vi "JSON Error to Error Cluster.vi"(8 "error in (no error)":errorcluster, 10 "headers":string, 11 "JSON string":string) -> (0 "error out":errorcluster)   [LabVIEW 2013, in "Particle API.lvlib"]
uses:
  Particle API.lvlib
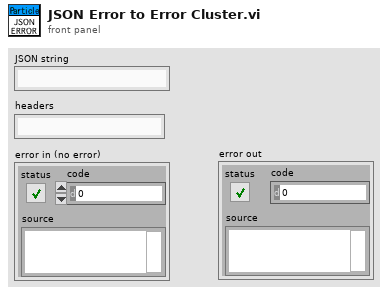
[diagram p1: front panel]
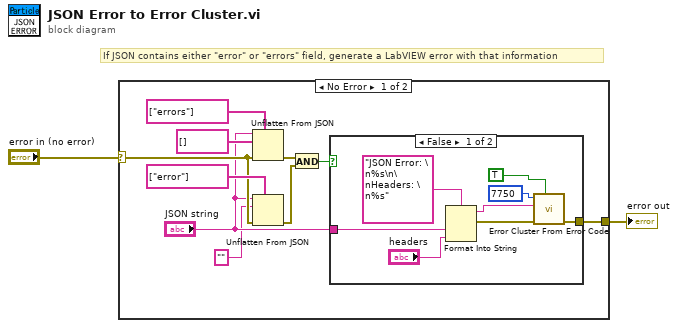
[diagram p0: block diagram]
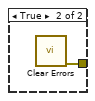
[diagram p2: hidden frame]
diagram:
  # "If JSON contains either \"error\" or \"errors\" field, generate a LabVIEW error with that information"
  n1 = case shown="No Error" "error in (no error)" {
    selector: "error in (no error)" -> [w8 w22]
    tunnel: [w12 w22] -> w1
    frame No Error {
      n2 = Unflatten From JSON(path=string[] ["errors"], JSON string="JSON string", type and defaults=string[] [], error in (no error)=w8) -> (error out=w5:errorcluster)  [unwired: 3 in, 1 out]
      n3 = Unflatten From JSON(path=string[] ["error"], JSON string="JSON string", type and defaults="", error in (no error)=w8) -> (error out=w4:errorcluster)  [unwired: 3 in, 1 out]
      n4 = And(x=w5, y=w4) -> (x .and. y?=w6:bool)
      n5 = case shown="False" w6 {
        tunnel: [w14 w21] -> w12
        tunnel: "JSON string" -> [w13 _]
        frame False {
          n6 = Format Into String(format string="JSON Error: \n%s\n\nHeaders: \n%s", w13, "headers") -> (resulting string=w17:string, error out=w16:errorcluster)  [unwired: 2 in]
          n7 = call <vilib>:"Error Cluster From Error Code.vi"("show call chain? (False)"=TRUE, "error in (no error)"=w16, "error message (\"\")"=w17, "error code (0)"=7750) -> ("error out"=w14:errorcluster)  [unwired: 5 in]
        }
        frame True {
          n8 = call <vilib>:"Clear Errors.vi"() -> ("error out"=w21:errorcluster)  [unwired: 7 in]
        }
      }
    }
    frame Error {
    }
  }
  "error out" <- w1
